vi "Camera_Feed.vi"(8 "error in":errorcluster, 11 "DataCluster":T1={"Core"={"Current VI Reference"=refnum, "Close Panel on Exit?"=FALSE, "Exit"=FALSE, "Initialized?"=FALSE}, "Connections"={"cDAQ"={"Task"="", "Connected"=FALSE, "Active"=FALSE, "ID"=""}, "Camera"={"Session"="", "Connected"=FALSE, "Active"=FALSE, "Placeholder"=refnum}, "PSU"={"Port"="", "Connected"=FALSE, "Active"=FALSE}, "Arduino"={"Port"="", "Connected"=FALSE, "Active"=FALSE}}, "Data Acquisition"={"Setup"={"Label"="", "Operator"="", "Notes"="", "TempGrad"=0.0, "TargetTemp"=0.0, "Sample Volume"=1.0}, "Camera"={"Image"=refnum, "Save Image"=refnum, "Image Frequency"=20, "Rectangle"={"Left"=0, "Top"=0, "Right"=0, "Bottom"=0, "Rotation"=0.0}, "Calibration"={"Top Left"={"X"=0.0, "Y"=0.0}, "Top Right"={"X"=0.0, "Y"=0.0}, "Bottom Left"={"X"=0.0, "Y"=0.0}, "Bottom Right"={"X"=0.0, "Y"=0.0}, "Fixpoint"={"X"=0.0, "Y"=0.0}, "Scan Area"=0.0, "Fixpoint Area"=0.0, "Well Pixels"=[], "Valid"=FALSE}, "FocusPos"=0, "Display Mapping"=10, "Camera Mode"=10}, "Thermistor"={"Sample Size"=0, "Calibration"={"B0.100"=[], "R25"=[], "c"=[], "State"=[], "V_S"=0.0, "R_S"=0.0}, "Timing Mode"=14713}, "Partition"={"Data"=[], "Cell Label"="", "Cell Color"=0, "Height"=10, "Width"=16, "Grid"=[]}, "Queue"={"Size"=0, "Queue"=refnum}, "Sample Rate"=0, "Active"=FALSE, "Ready"=FALSE, "Graph Mode"=0, "Gradient Buffer"=2}, "Control"={"Sample Rate"=0, "PID gains"={"proportional gain (Kc)"=0.0, "integral time (Ti, min)"=0.0, "derivative time (Td, min)"=0.0}}, "Manual Temp Control"={"TargetTemp"=1.0, "Mode"=0, "Active"=FALSE}} {"Manual Temp Control"."Mode" items=["Cool", "Heat"]; "Manual Temp Control"."TargetTemp" min=-40.0 max=40.0 step=0.5 format="%#_g °C"; "Control"."PID gains"."derivative time (Td, min)" format="%.3f"; "Control"."PID gains"."integral time (Ti, min)" format="%.3f"; "Control"."PID gains"."proportional gain (Kc)" format="%.3f"; "Control"."Sample Rate" min=1 max=20 step=1 format="%.0f Samples/sec"; "Data Acquisition"."Gradient Buffer" min=2 max=30 step=1; "Data Acquisition"."Graph Mode" items=["Thermistor Temperature", "Camera Temperature"]; "Data Acquisition"."Thermistor"."Timing Mode" items=["Automatic"=16097, "High Resolution"=10195, "High Speed"=14712, "Best 50 Hz Rejection"=14713, "Best 60 Hz Rejection"=14714, "Custom"=10137]; "Data Acquisition"."Thermistor"."Calibration"."R_S" min=0.1 max=1000.0 format="%#_g kOhm"; "Data Acquisition"."Thermistor"."Calibration"."V_S" min=5.0 max=48.0 format="%#_g V"; "Data Acquisition"."Thermistor"."Calibration"."R25" min=0.1 max=1000.0 format="%#_g kOhm"; "Data Acquisition"."Thermistor"."Calibration"."B0.100" min=100.0 max=10000.0 format="%#_g K"; "Data Acquisition"."Thermistor"."Sample Size" min=1 max=200; "Data Acquisition"."Sample Rate" min=20 max=240 format="%.0f samples/min"; "Data Acquisition"."Queue"."Size" min=1 max=200; "Data Acquisition"."Camera"."Camera Mode" items=["Temperature Linear", "Signal Linear"]; "Data Acquisition"."Camera"."Display Mapping" items=["Default"=10, "Most Significant Bits"=11, "Full Dynamic"=12, "Downshift"=13, "Given Range"=14, "90% Dynamic"=15, "Given Percent Range"=16]; "Data Acquisition"."Camera"."Calibration"."Fixpoint"."Y" format="%.2f"; "Data Acquisition"."Camera"."Calibration"."Fixpoint"."X" format="%.2f"; "Data Acquisition"."Camera"."Calibration"."Top Left"."Y" format="%.2f"; "Data Acquisition"."Camera"."Calibration"."Top Left"."X" format="%.2f"; "Data Acquisition"."Camera"."Calibration"."Top Right"."Y" format="%.2f"; "Data Acquisition"."Camera"."Calibration"."Top Right"."X" format="%.2f"; "Data Acquisition"."Camera"."Calibration"."Bottom Left"."Y" format="%.2f"; "Data Acquisition"."Camera"."Calibration"."Bottom Left"."X" format="%.2f"; "Data Acquisition"."Camera"."Calibration"."Bottom Right"."Y" format="%.2f"; "Data Acquisition"."Camera"."Calibration"."Bottom Right"."X" format="%.2f"; "Data Acquisition"."Camera"."Rectangle"."Rotation" min=-90.0 max=90.0 step=1.0 format="%.2f"; "Data Acquisition"."Camera"."Rectangle"."Left" scale=0.0..1024.0; "Data Acquisition"."Camera"."Rectangle"."Right" scale=0.0..1024.0; "Data Acquisition"."Camera"."Image Frequency" min=1 max=60 step=1; "Data Acquisition"."Setup"."Sample Volume" min=0.0 max=500.0 format="%#_g µL"; "Data Acquisition"."Setup"."TargetTemp" min=-40.0 max=40.0 step=0.5 format="%#_g °C"; "Data Acquisition"."Setup"."TempGrad" min=-100.0 max=100.0 step=0.1 format="%#_g °C/min"}) -> (0 "error out":errorcluster, 3 "DataCluster out":T1={"Core"={"Current VI Reference"=refnum, "Close Panel on Exit?"=FALSE, "Exit"=FALSE, "Initialized?"=FALSE}, "Connections"={"cDAQ"={"Task"="", "Connected"=FALSE, "Active"=FALSE, "ID"=""}, "Camera"={"Session"="", "Connected"=FALSE, "Active"=FALSE, "Placeholder"=refnum}, "PSU"={"Port"="", "Connected"=FALSE, "Active"=FALSE}, "Arduino"={"Port"="", "Connected"=FALSE, "Active"=FALSE}}, "Data Acquisition"={"Setup"={"Label"="", "Operator"="", "Notes"="", "TempGrad"=1.0, "TargetTemp"=1.0, "Sample Volume"=1.0}, "Camera"={"Image"=refnum, "Save Image"=refnum, "Image Frequency"=20, "Rectangle"={"Left"=0, "Top"=0, "Right"=0, "Bottom"=0, "Rotation"=0.0}, "Calibration"={"Top Left"={"X"=0.0, "Y"=0.0}, "Top Right"={"X"=0.0, "Y"=0.0}, "Bottom Left"={"X"=0.0, "Y"=0.0}, "Bottom Right"={"X"=0.0, "Y"=0.0}, "Fixpoint"={"X"=0.0, "Y"=0.0}, "Scan Area"=0.0, "Fixpoint Area"=0.0, "Well Pixels"=[], "Valid"=FALSE}, "FocusPos"=0, "Display Mapping"=10, "Camera Mode"=10}, "Thermistor"={"Sample Size"=1, "Calibration"={"B0.100"=[], "R25"=[], "c"=[], "State"=[], "V_S"=5.0, "R_S"=100.0}, "Timing Mode"=14713}, "Partition"={"Data"=[], "Cell Label"="", "Cell Color"=0, "Height"=10, "Width"=16, "Grid"=[]}, "Queue"={"Size"=1, "Queue"=refnum}, "Sample Rate"=20, "Active"=FALSE, "Ready"=FALSE, "Graph Mode"=0, "Gradient Buffer"=2}, "Control"={"Sample Rate"=1, "PID gains"={"proportional gain (Kc)"=1.0, "integral time (Ti, min)"=0.01, "derivative time (Td, min)"=0.0}}, "Manual Temp Control"={"TargetTemp"=1.0, "Mode"=0, "Active"=FALSE}} {"Manual Temp Control"."Mode" items=["Cool", "Heat"]; "Manual Temp Control"."TargetTemp" min=-40.0 max=40.0 step=0.5 format="%#_g °C"; "Control"."PID gains"."derivative time (Td, min)" format="%.3f"; "Control"."PID gains"."integral time (Ti, min)" format="%.3f"; "Control"."PID gains"."proportional gain (Kc)" format="%.3f"; "Control"."Sample Rate" min=1 max=20 step=1 format="%.0f Samples/sec"; "Data Acquisition"."Gradient Buffer" min=2 max=30 step=1; "Data Acquisition"."Graph Mode" items=["Thermistor Temperature", "Camera Temperature"]; "Data Acquisition"."Thermistor"."Timing Mode" items=["Automatic"=16097, "High Resolution"=10195, "High Speed"=14712, "Best 50 Hz Rejection"=14713, "Best 60 Hz Rejection"=14714, "Custom"=10137]; "Data Acquisition"."Thermistor"."Calibration"."R_S" min=0.1 max=1000.0 format="%#_g kOhm"; "Data Acquisition"."Thermistor"."Calibration"."V_S" min=5.0 max=48.0 format="%#_g V"; "Data Acquisition"."Thermistor"."Calibration"."R25" min=0.1 max=1000.0 format="%#_g kOhm"; "Data Acquisition"."Thermistor"."Calibration"."B0.100" min=100.0 max=10000.0 format="%#_g K"; "Data Acquisition"."Thermistor"."Sample Size" min=1 max=200; "Data Acquisition"."Sample Rate" min=20 max=240 format="%.0f samples/min"; "Data Acquisition"."Queue"."Size" min=1 max=200; "Data Acquisition"."Camera"."Camera Mode" items=["Temperature Linear", "Signal Linear"]; "Data Acquisition"."Camera"."Display Mapping" items=["Default"=10, "Most Significant Bits"=11, "Full Dynamic"=12, "Downshift"=13, "Given Range"=14, "90% Dynamic"=15, "Given Percent Range"=16]; "Data Acquisition"."Camera"."Calibration"."Fixpoint"."Y" format="%.2f"; "Data Acquisition"."Camera"."Calibration"."Fixpoint"."X" format="%.2f"; "Data Acquisition"."Camera"."Calibration"."Top Left"."Y" format="%.2f"; "Data Acquisition"."Camera"."Calibration"."Top Left"."X" format="%.2f"; "Data Acquisition"."Camera"."Calibration"."Top Right"."Y" format="%.2f"; "Data Acquisition"."Camera"."Calibration"."Top Right"."X" format="%.2f"; "Data Acquisition"."Camera"."Calibration"."Bottom Left"."Y" format="%.2f"; "Data Acquisition"."Camera"."Calibration"."Bottom Left"."X" format="%.2f"; "Data Acquisition"."Camera"."Calibration"."Bottom Right"."Y" format="%.2f"; "Data Acquisition"."Camera"."Calibration"."Bottom Right"."X" format="%.2f"; "Data Acquisition"."Camera"."Rectangle"."Rotation" min=-90.0 max=90.0 step=1.0 format="%.2f"; "Data Acquisition"."Camera"."Rectangle"."Left" scale=0.0..1024.0; "Data Acquisition"."Camera"."Rectangle"."Right" scale=0.0..1024.0; "Data Acquisition"."Camera"."Image Frequency" min=1 max=60 step=1; "Data Acquisition"."Setup"."Sample Volume" min=0.0 max=500.0 format="%#_g µL"; "Data Acquisition"."Setup"."TargetTemp" min=-40.0 max=40.0 step=0.5 format="%#_g °C"; "Data Acquisition"."Setup"."TempGrad" min=-100.0 max=100.0 step=0.1 format="%#_g °C/min"})   [LabVIEW 2024]
uses:
  DataCluster.ctl
  <vilib>/userDefined/High Color/IMAQdx.ctl
  <vilib>/vision/Image Controls.llb/IMAQ Image.ctl
  <resource>/objmgr/imaqdx.rc
panel:
  out "Feed":T3(plugin-control) caption="Camera Feed"
  out "CameraModeDesc":string
  in  "Camera Mode":u32(ring)=10 items=["Temperature Linear", "Radiometric"]
  out "FocusPos":u32 caption="Focus Position"
  in  "Autofocus":bool
  in  "Cropping":enum32{"Cropped", "Uncropped"}(radio)=enum."Uncropped"
  out "StatusString":string="Closing System"
  # "Select Region of Interest on the camera feed and see the  cropped image by selecting Cropped.\n\nMake sure the entire plate is within the boundaries"
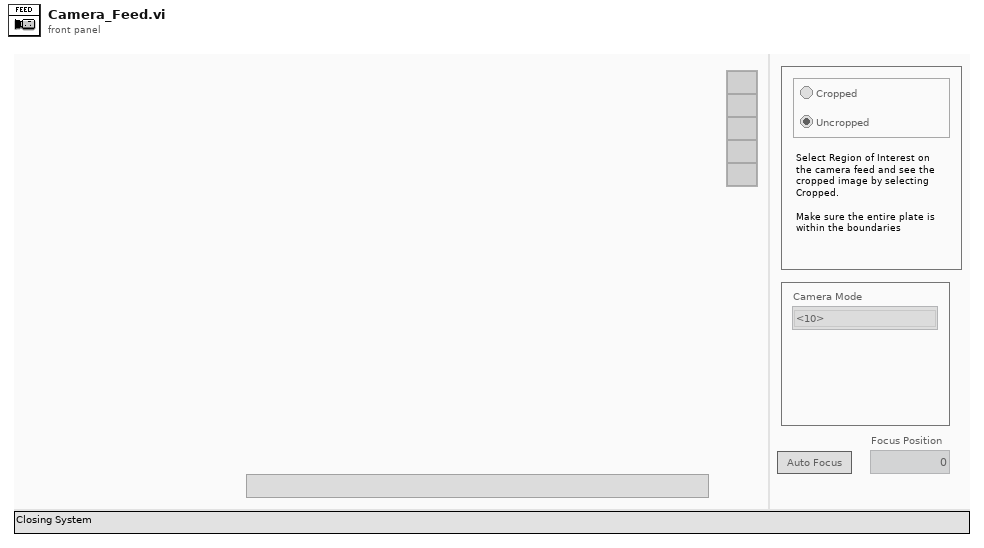
[diagram p1: front panel]
types:
  T1 = typedef "DataCluster.ctl" = cluster{"Core":cluster{"Current VI Reference":refnum<vi>, "Close Panel on Exit?":bool, "Exit":bool, "Initialized?":bool}, "Connections":cluster{"cDAQ":cluster{"Task":refnum<k21>, "Connected":bool, "Active":bool, "ID":string}, "Camera":cluster{"Session":T2, "Connected":bool, "Active":bool, "Placeholder":T3}, "PSU":cluster{"Port":refnum<visa-resource-name>, "Connected":bool, "Active":bool}, "Arduino":cluster{"Port":refnum<visa-resource-name>, "Connected":bool, "Active":bool}}, "Data Acquisition":cluster{"Setup":cluster{"Label":string, "Operator":string, "Notes":string, "TempGrad":dbl, "TargetTemp":dbl, "Sample Volume":dbl}, "Camera":cluster{"Image":T3, "Save Image":T3, "Image Frequency":i32, "Rectangle":T4, "Calibration":cluster{"Top Left":T5, "Top Right":T5, "Bottom Left":T5, "Bottom Right":T5, "Fixpoint":T5, "Scan Area":dbl, "Fixpoint Area":dbl, "Well Pixels":cluster{"X":i32, "Y":i32}[][], "Valid":bool}, "FocusPos":u32, "Display Mapping":u32, "Camera Mode":u32}, "Thermistor":cluster{"Sample Size":i32, "Calibration":cluster{"B0.100":dbl[], "R25":dbl[], "c":dbl[][], "State":bool[], "V_S":dbl, "R_S":dbl}, "Timing Mode":i32}, "Partition":cluster{"Data":string[][], "Cell Label":string, "Cell Color":u32, "Height":i32, "Width":i32, "Grid":string[][]}, "Queue":cluster{"Size":i32, "Queue":refnum<queue>}, "Sample Rate":i32, "Active":bool, "Ready":bool, "Graph Mode":u16, "Gradient Buffer":i32}, "Control":cluster{"Sample Rate":i32, "PID gains":cluster{"proportional gain (Kc)":dbl, "integral time (Ti, min)":dbl, "derivative time (Td, min)":dbl}}, "Manual Temp Control":cluster{"TargetTemp":dbl, "Mode":u16, "Active":bool}}
  T2 = typedef "IMAQdx.ctl" = refnum<k21>
  T3 = typedef "IMAQ Image.ctl" = refnum<image>
  T4 = typedef "IMAQ Rectangle" = cluster{"Left":i32, "Top":i32, "Right":i32, "Bottom":i32, "Rotation":dbl}
  T5 = typedef "IMAQ Point" = cluster{"X":sgl, "Y":sgl}
  T6 = enum32{"Invalid", "Standard", "Closed", "Hidden", "Minimized", "Maximized"}
  T7 = enum8{"Enabled", "Disabled", "Disabled and Grayed Out"}
  T8 = cluster{"Global Rectangle":i32[], "Contours":cluster{"Contour Type":u32, "ROI Type":u32, "Points":i32[]}[]}
  T9 = typedef "ROI Descriptor" = cluster{"Global Rectangle":i32[], "Contours":cluster{"ID":enum32{"External", "Internal"}, "Type":u32, "Coordinates":i32[]}[]}
  T10 = cluster{"Global Rectangle":i32[], "Contours":cluster{"Contour Type":u32, "Type":u32, "Coordinates":i32[]}[]}
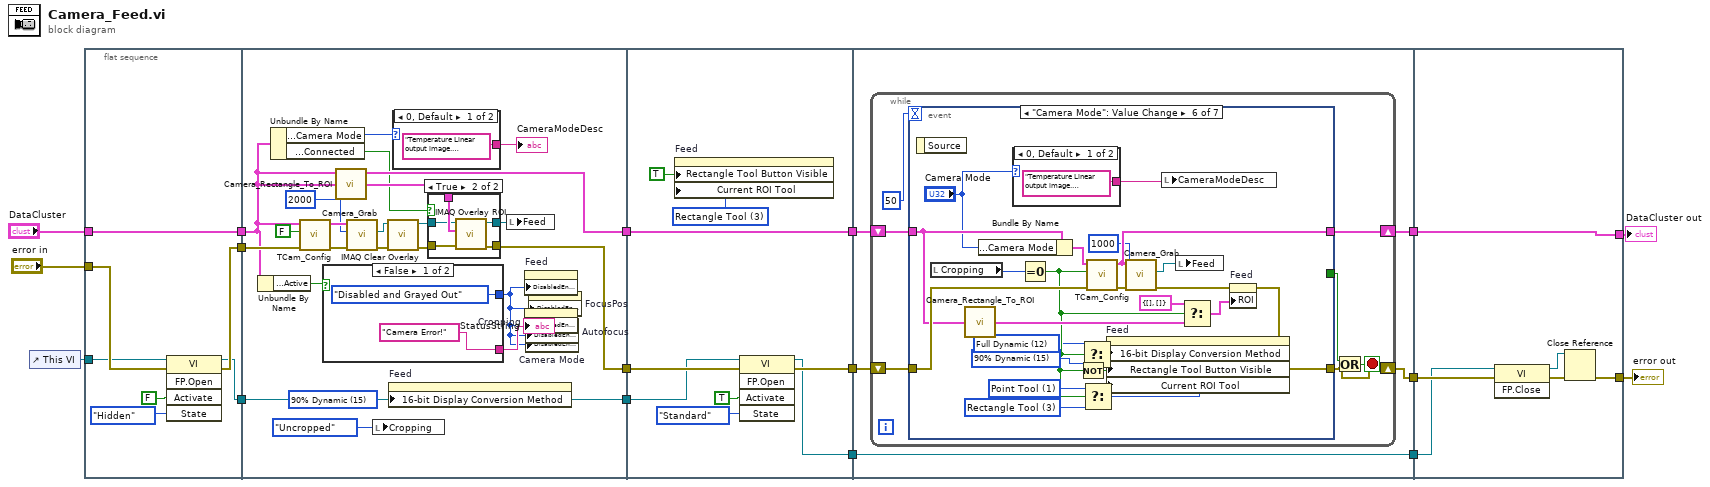
[diagram p0: block diagram]
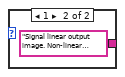
[diagram p2: hidden frame]
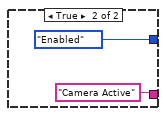
[diagram p4: hidden frame]
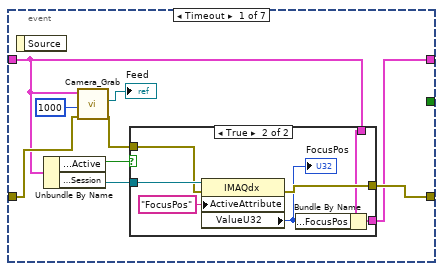
[diagram p5: hidden frame]
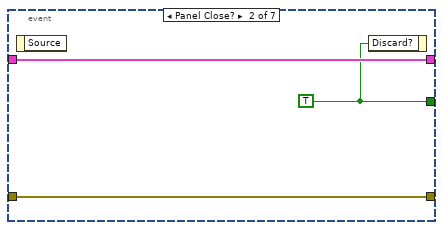
[diagram p7: hidden frame]
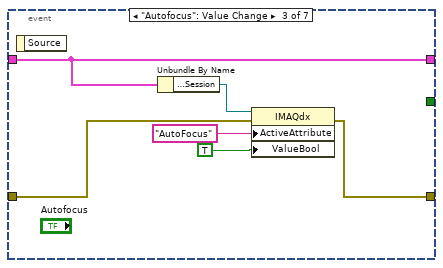
[diagram p8: hidden frame]
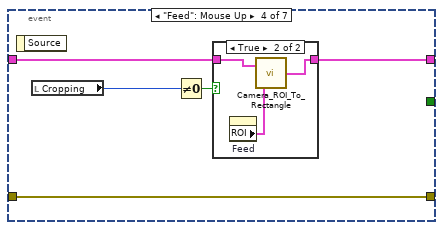
[diagram p9: hidden frame]
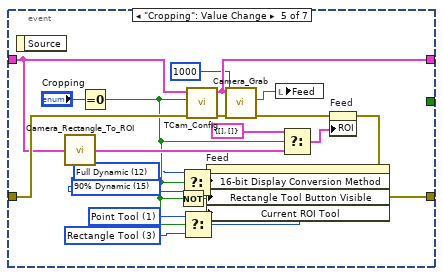
[diagram p11: hidden frame]
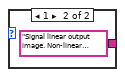
[diagram p12: hidden frame]
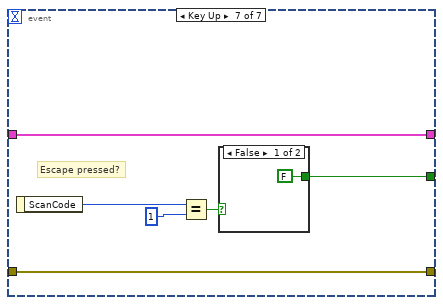
[diagram p13: hidden frame]
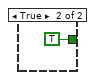
[diagram p14: hidden frame]
diagram:
  n1 = control-ref of="This VI"() -> (w3:refnum<vi>)
  n2 = flat-sequence {
    tunnel: "DataCluster" -> [w24]
    tunnel: "error in" -> [w23]
    tunnel: [w24] -> w7
    tunnel: w3 -> [w22]
    tunnel: [w20] -> w6
    tunnel: [w19] -> w4
    tunnel: [w40] -> w11
    tunnel: [w34] -> w9
    tunnel: w7 -> [w34]
    tunnel: w6 -> [w39]
    tunnel: [w38] -> w5
    tunnel: w4 -> [w38]
    tunnel: w11 -> [w65]
    tunnel: [w63] -> w10
    tunnel: w9 -> [w68]
    tunnel: [w68] -> w8
    tunnel: w5 -> [w64]
    tunnel: [w62] -> w1
    tunnel: [w71] -> w14
    tunnel: w10 -> [w73]
    tunnel: [w70] -> w13
    tunnel: w8 -> [w72]
    tunnel: [w69] -> w2
    tunnel: w1 -> [w69]
    tunnel: [w172] -> w15
    tunnel: w14 -> [w171]
    tunnel: [w175] -> w12
    tunnel: w13 -> [w175]
    tunnel: w2 -> [w170]
    frame #0 {
      n3 = invoke class="VI" method="FP.Open"(reference=w22, error in=w23, "Activate"=FALSE ("Activate?"), "State"=T6."Hidden") -> (reference out=w19:refnum<vi>, error out=w20:errorcluster)  [unwired: 1 in, 3 out]
    }
    frame #1 {
      w32 = u32 15 items=["Default"=10, "Most Significant Bits"=11, "Full Dynamic"=12, "Downshift"=13, "Given Range"=14, "90% Dynamic"=15, "Given Percent Range"=16] ("16-bit Display Mapping:Conversion Method")
      n4 = Unbundle By Name(w34) -> ("Connections.Camera.Active"=w45:bool)
      n5 = Unbundle By Name(w34) -> ("Data Acquisition.Camera.Camera Mode"=w26:u32, "Connections.Camera.Connected"=w33:bool)
      n6 = call "TCam_Config.vi"("error in (no error)"=w39, "crop?"=FALSE, "DataCluster in"=w34) -> ("error out"=w41:errorcluster, "DataCluster out"=w42:T1)  [unwired: 7 in]
      n7 = case shown="False" w45 {
        tunnel: [T7."Disabled and Grayed Out" ("Disabled") T7."Enabled" ("Disabled")] -> w27
        tunnel: ["Camera Error!" "Camera Active"] -> w44
        frame False {
        }
        frame True {
        }
      }
      "StatusString" <- w44
      n8 = call "Camera_Rectangle_To_ROI.vi"("input cluster"=w34) -> ("ROI Descriptor"=w36:T9)
      n9 = call "Camera_Grab.vi"("error in"=w41, "Timeout (ms)"=2000, "DataCluster"=w42) -> ("error out"=w31:errorcluster, "Image Out"=w28:T3)  [unwired: 6 in, 1 out]
      n10 = local write "Cropping"(enum32{"Cropped", "Uncropped"}."Uncropped" ("Cropping")) -> ()
      n11 = call "IMAQ Clear Overlay"("error in (no error)"=w31, "Image"=w28) -> ("error out"=w30:errorcluster, "Image Out"=w29:T3)  [unwired: 8 in]
      n12 = property on="Feed" class="ImageControl"("16-bit Display Conversion Method"=w32) -> ()  [unwired: 2 in, 2 out]
      n13 = case shown="0, Default" w26 {
        tunnel: ["Temperature Linear output image. Temperature conversion calculations handled by camera. " "Signal linear output image. Non-linear temperature calculations needed in post processing."] -> w25
        frame 0, Default {
        }
        frame 1 {
        }
      }
      "CameraModeDesc" <- w25
      n14 = case shown="True" w33 {
        tunnel: w29 -> [w49 w51]
        tunnel: w30 -> [w50 w52]
        tunnel: [w50 w55] -> w40
        tunnel: w36 -> [_ w54]
        tunnel: [w49 w53] -> w35
        frame False {
        }
        frame True {
          n15 = call "IMAQ Overlay ROI"("error in (no error)"=w52, "ROI Descriptor"=w54, "Image"=w51) -> ("error out"=w55:errorcluster, "Image Out"=w53:T3)  [unwired: 7 in]
        }
      }
      n16 = local write "Feed"(w35) -> ()
      n17 = property on="Feed" class="ImageControl"("DisabledEnum"=w27) -> ()  [unwired: 2 in, 2 out]
      n18 = property on="Cropping" class="RadioBtnsControl (strict)"("DisabledEnum"=w27) -> ()  [unwired: 2 in, 2 out]
      n19 = property on="Autofocus" class="Bool"("DisabledEnum"=w27) -> ()  [unwired: 2 in, 2 out]
      n20 = property on="Camera Mode" class="Ring (strict)"("DisabledEnum"=w27) -> ()  [unwired: 2 in, 2 out]
      n21 = property on="FocusPos" class="DigNum (strict)"("DisabledEnum"=w27) -> ()  [unwired: 2 in, 2 out]
    }
    frame #2 {
      w60 = u32 3 items=["Zoom Tool"=8, "Selection Tool"=0, "Pan Tool"=9, "Point Tool"=1, "Line Tool"=2, "Rectangle Tool"=3, "Rotated Rectangle Tool"=12, "Polyline Tool"=10, "Polygon Tool"=5, "Freehand Tool"=11, "Closed Freehand Tool"=6, "Ellipse Tool"=4, "Annulus Tool"=7] ("Current ROI Tool")
      n22 = property on="Feed" class="ImageControl"("Rectangle Tool Button Visible"=TRUE ("ROI Tool Buttons Visible:Rectangle Tool Button Visible"), "Current ROI Tool"=w60) -> ()  [unwired: 2 in, 2 out]
      n23 = invoke class="VI" method="FP.Open"(reference=w64, error in=w65, "Activate"=TRUE ("Activate?"), "State"=T6."Standard") -> (reference out=w62:refnum<vi>, error out=w63:errorcluster)  [unwired: 1 in, 3 out]
    }
    frame #3 {
      n24 = while {
        shift-right: [w78] -> w70
        shift-left: w72 -> [w77]
        shift-right: [w75] -> w71
        shift-left: w73 -> [w76]
        stop <- w79 stop-if-true
        n25 = event shown="[5] \"Camera Mode\": Value Change" {
          selector: _ -> [_ _ _ _ _ _ _]
          dyn-events: _ -> [_ _ _ _ _ _ _]
          timeout: 50 -> [_ _ _ _ _ _ _]
          tunnel: [_ w99 _ _ _ _ w167] -> w80
          tunnel: [w83 w101 w105 w112 w130 w154 w163] -> w78
          tunnel: w77 -> [w84 w101 w105 w109 w128 w152 w163]
          tunnel: w76 -> [w89 w100 w103 w108 w135 w159 w162]
          tunnel: [w85 w100 w102 w108 w132 w156 w162] -> w75
          event Timeout {
            n26 = event-data() -> ()  [unwired: 1 in, 1 out]
            n27 = Unbundle By Name(w84) -> ("Connections.Camera.Active"=w82:bool, "Connections.Camera.Session"=w87:T2)
            n28 = call "Camera_Grab.vi"("error in"=w89, "Timeout (ms)"=1000, "DataCluster"=w84) -> ("error out"=w86:errorcluster, "Image Out"=→"Feed":T3)  [unwired: 6 in, 1 out]
            n29 = case shown="True" w82 {
              tunnel: w87 -> [_ w97]
              tunnel: w86 -> [w91 w96]
              tunnel: [w91 w95] -> w85
              tunnel: w84 -> [w90 w94]
              tunnel: [w90 w93] -> w83
              frame False {
              }
              frame True {
                n30 = property class="IMAQdx"(reference=w97, error in=w96, "ActiveAttribute"="FocusPos") -> (error out=w95:errorcluster, "ValueU32"=w92:u32)  [unwired: 1 out]
                "FocusPos" <- w92
                n31 = Bundle By Name(cluster=w94, "Data Acquisition.Camera.FocusPos"=w92) -> (w93:T1)
              }
            }
          }
          event Panel Close? {
            w99 = TRUE
            n32 = event-data() -> ()  [unwired: 1 in, 1 out]
            n33 = event-data("Discard?"=w99) -> ()  [unwired: 1 in, 1 out]
          }
          event "Autofocus": Value Change {
            n34 = event-data() -> ()  [unwired: 1 in, 1 out]
            n35 = Unbundle By Name(w105) -> ("Connections.Camera.Session"=w104:T2)
            n36 = property class="IMAQdx"(reference=w104, error in=w103, "ActiveAttribute"="AutoFocus", "ValueBool"=TRUE) -> (error out=w102:errorcluster)  [unwired: 1 out]
          }
          event "Feed": Mouse Up {
            n37 = event-data() -> ()  [unwired: 1 in, 1 out]
            n38 = local read "Cropping"() -> (w111:enum32{"Cropped", "Uncropped"})
            n39 = Not Equal To 0?(x=w111) -> (x != 0?=w110:bool)
            n40 = case shown="True" w110 {
              tunnel: [w113 w115] -> w112
              tunnel: w109 -> [w113 w116]
              frame False {
              }
              frame True {
                n41 = property on="Feed" class="ImageControl"() -> ("ROI"=w114:T8)  [unwired: 2 in, 2 out]
                n42 = call "Camera_ROI_To_Rectangle.vi"("ROI Descriptor"=w114, "input cluster"=w116) -> ("output cluster"=w115:T1)
              }
            }
          }
          event "Cropping": Value Change {
            w118 = u32 12 items=["Default"=10, "Most Significant Bits"=11, "Full Dynamic"=12, "Downshift"=13, "Given Range"=14, "90% Dynamic"=15, "Given Percent Range"=16] ("16-bit Display Mapping:Conversion Method")
            w119 = u32 15 items=["Default"=10, "Most Significant Bits"=11, "Full Dynamic"=12, "Downshift"=13, "Given Range"=14, "90% Dynamic"=15, "Given Percent Range"=16] ("16-bit Display Mapping:Conversion Method")
            w122 = u32 3 items=["Zoom Tool"=8, "Selection Tool"=0, "Pan Tool"=9, "Point Tool"=1, "Line Tool"=2, "Rectangle Tool"=3, "Rotated Rectangle Tool"=12, "Polyline Tool"=10, "Polygon Tool"=5, "Freehand Tool"=11, "Closed Freehand Tool"=6, "Ellipse Tool"=4, "Annulus Tool"=7] ("Current ROI Tool")
            w124 = u32 1 items=["Zoom Tool"=8, "Selection Tool"=0, "Pan Tool"=9, "Point Tool"=1, "Line Tool"=2, "Rectangle Tool"=3, "Rotated Rectangle Tool"=12, "Polyline Tool"=10, "Polygon Tool"=5, "Freehand Tool"=11, "Closed Freehand Tool"=6, "Ellipse Tool"=4, "Annulus Tool"=7] ("Current ROI Tool")
            n43 = event-data() -> ()  [unwired: 1 in, 1 out]
            n44 = call "Camera_Rectangle_To_ROI.vi"("input cluster"=w128) -> ("ROI Descriptor"=w127:T9)
            n45 = Equal To 0?(x="Cropping") -> (x = 0?=w120:bool)
            n46 = Not(x=w120) -> (.not. x?=w125:bool)
            n47 = Select(t=w118, s=w120, f=w119) -> (s? t:f=w121:u32)
            n48 = Select(t=w124, s=w120, f=w122) -> (s? t:f=w123:u32)
            n49 = call "TCam_Config.vi"("error in (no error)"=w135, "crop?"=w120, "DataCluster in"=w128) -> ("error out"=w131:errorcluster, "DataCluster out"=w130:T1)  [unwired: 7 in]
            n50 = property on="Feed" class="ImageControl"("16-bit Display Conversion Method"=w121, "Rectangle Tool Button Visible"=w125, "Current ROI Tool"=w123) -> ()  [unwired: 2 in, 2 out]
            n51 = call "Camera_Grab.vi"("error in"=w131, "Timeout (ms)"=1000, "DataCluster"=w130) -> ("error out"=w126:errorcluster, "Image Out"=w117:T3)  [unwired: 6 in, 1 out]
            n52 = local write "Feed"(w117) -> ()
            n53 = Select(t=T8 {"Global Rectangle"=[], "Contours"=[]} ("ROI"), s=w120, f=w127) -> (s? t:f=w134:T10)
            n54 = property on="Feed" class="ImageControl"(error in=w126, "ROI"=w134) -> (error out=w132:errorcluster)  [unwired: 1 in, 1 out]
          }
          event "Camera Mode": Value Change {
            w142 = u32 12 items=["Default"=10, "Most Significant Bits"=11, "Full Dynamic"=12, "Downshift"=13, "Given Range"=14, "90% Dynamic"=15, "Given Percent Range"=16] ("16-bit Display Mapping:Conversion Method")
            w143 = u32 15 items=["Default"=10, "Most Significant Bits"=11, "Full Dynamic"=12, "Downshift"=13, "Given Range"=14, "90% Dynamic"=15, "Given Percent Range"=16] ("16-bit Display Mapping:Conversion Method")
            w146 = u32 3 items=["Zoom Tool"=8, "Selection Tool"=0, "Pan Tool"=9, "Point Tool"=1, "Line Tool"=2, "Rectangle Tool"=3, "Rotated Rectangle Tool"=12, "Polyline Tool"=10, "Polygon Tool"=5, "Freehand Tool"=11, "Closed Freehand Tool"=6, "Ellipse Tool"=4, "Annulus Tool"=7] ("Current ROI Tool")
            w148 = u32 1 items=["Zoom Tool"=8, "Selection Tool"=0, "Pan Tool"=9, "Point Tool"=1, "Line Tool"=2, "Rectangle Tool"=3, "Rotated Rectangle Tool"=12, "Polyline Tool"=10, "Polygon Tool"=5, "Freehand Tool"=11, "Closed Freehand Tool"=6, "Ellipse Tool"=4, "Annulus Tool"=7] ("Current ROI Tool")
            n55 = event-data() -> ()  [unwired: 1 in, 1 out]
            n56 = local read "Cropping"() -> (w140:enum32{"Cropped", "Uncropped"})
            n57 = call "Camera_Rectangle_To_ROI.vi"("input cluster"=w152) -> ("ROI Descriptor"=w151:T9)
            n58 = Bundle By Name(cluster=w152, "Data Acquisition.Camera.Camera Mode"="Camera Mode") -> (w139:T1)
            n59 = case shown="0, Default" "Camera Mode" {
              tunnel: ["Temperature Linear output image. Temperature conversion calculations handled by camera. " "Signal linear output image. Non-linear temperature calculations needed in post processing."] -> w137
              frame 0, Default {
              }
              frame 1 {
              }
            }
            n60 = Equal To 0?(x=w140) -> (x = 0?=w144:bool)
            n61 = Not(x=w144) -> (.not. x?=w149:bool)
            n62 = Select(t=w142, s=w144, f=w143) -> (s? t:f=w145:u32)
            n63 = Select(t=w148, s=w144, f=w146) -> (s? t:f=w147:u32)
            n64 = call "TCam_Config.vi"("error in (no error)"=w159, "crop?"=w144, "DataCluster in"=w139) -> ("error out"=w155:errorcluster, "DataCluster out"=w154:T1)  [unwired: 7 in]
            n65 = property on="Feed" class="ImageControl"("16-bit Display Conversion Method"=w145, "Rectangle Tool Button Visible"=w149, "Current ROI Tool"=w147) -> ()  [unwired: 2 in, 2 out]
            n66 = call "Camera_Grab.vi"("error in"=w155, "Timeout (ms)"=1000, "DataCluster"=w154) -> ("error out"=w150:errorcluster, "Image Out"=w141:T3)  [unwired: 6 in, 1 out]
            n67 = local write "CameraModeDesc"(w137) -> ()
            n68 = local write "Feed"(w141) -> ()
            n69 = Select(t=T8 {"Global Rectangle"=[], "Contours"=[]} ("ROI"), s=w144, f=w151) -> (s? t:f=w158:T10)
            n70 = property on="Feed" class="ImageControl"(error in=w150, "ROI"=w158) -> (error out=w156:errorcluster)  [unwired: 1 in, 1 out]
          }
          event Key Up {
            # "Escape pressed?"
            n71 = event-data() -> ("ScanCode"=w166:i16)  [unwired: 1 in]
            n72 = Equal?(x=w166, y=i16 1) -> (x = y?=w164:bool)
            n73 = case shown="False" w164 {
              tunnel: [FALSE TRUE] -> w167
              frame False {
              }
              frame True {
              }
            }
          }
        }
        n74 = Or(x=w80, y=w75) -> (x .or. y?=w79:bool)
      }
    }
    frame #4 {
      n75 = invoke class="VI" method="FP.Close"(reference=w170, error in=w171) -> (reference out=w174:refnum<vi>, error out=w173:errorcluster)  [unwired: 1 in, 1 out]
      n76 = Close Reference(reference=w174, error in (no error)=w173) -> (error out=w172:errorcluster)
    }
  }
  "error out" <- w15
  "DataCluster out" <- w12
